vi "SW_Check_segments_parameters_2.vi"(3 "Error In":errorcluster, 5 "Geometry in":T1 {"Cage type" items=["Round", "Square", "Donut-maze", "T-maze", "Sociability maze", ""]}) -> (0 "Error Out":errorcluster, 1 "Segmentation out":T4={"CENTER"={"Radius, mm CENTER"=30}, "MIDFIELD"={"Radius, mm MIDFIELD"=75, "N segments MIDFIELD"=2, "Starting angle MIDFIELD"=0}, "BORDER"={"N segments BORDER"=4, "Starting angle BORDER"=0}} {"BORDER"."N segments BORDER" min=1 max=12; "MIDFIELD"."N segments MIDFIELD" max=8; "CENTER"."Radius, mm CENTER" min=5 step=1}, 2 "Geometry out":T1 {"Cage type" items=["Round", "Square", "Donut-maze", "T-maze", "Sociability maze", ""]})   [LabVIEW 2018, in "Tracker.lvlib"]
uses:
  Tracker.lvlib
  Controls/CTL_Cage_radial_segmentation.ctl
  Controls/CTL_Segmented_plot_parameters_2.ctl
  Libraries/Cage Diagram/Typedefs/CTL_Cage_type.ctl
  Controls/CTL_Cage_all_segmentation_params_set.ctl
  Controls/CTL_Segmented_plot_parameters_2_(round_d1).ctl
  Common_Resources.lvlib
  Libraries/Cage Diagram/Cage Diagram.lvlib
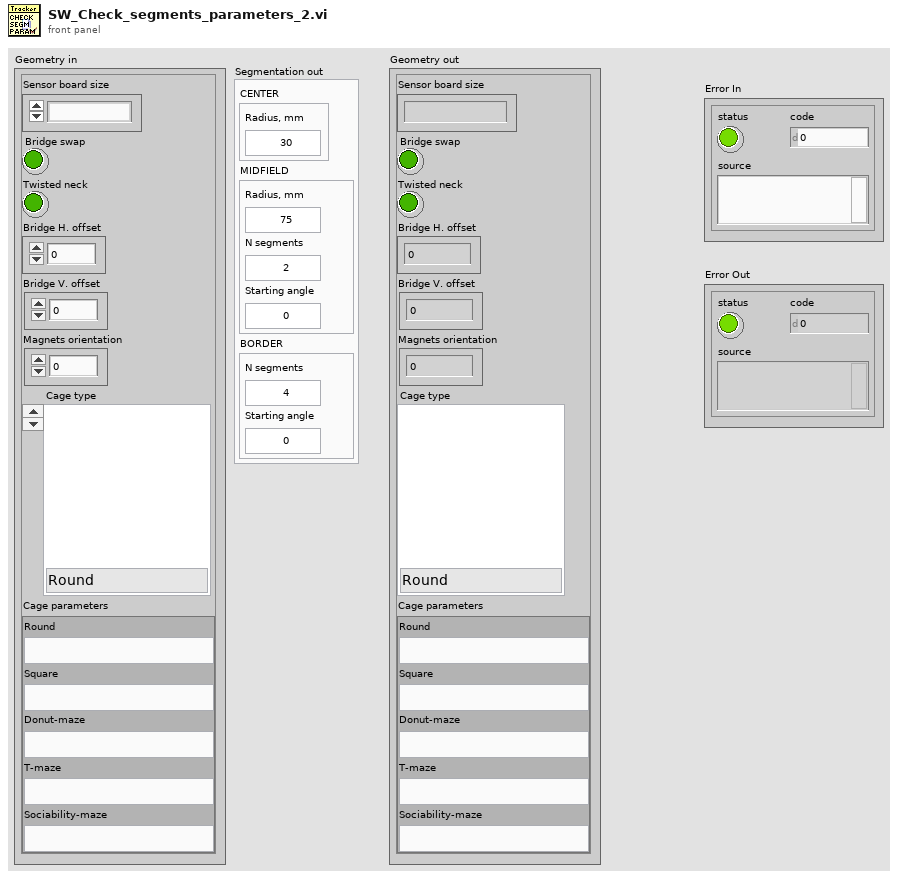
[diagram p1: front panel]
types:
  T1 = typedef "Common_Resources.lvlib/CTL_Segmented_plot_parameters_2.ctl" = cluster{"Sensor board size":enum16{"", "Large"}, "Bridge swap":bool, "Twisted neck":bool, "Bridge H. offset":sgl, "Bridge V. offset":sgl, "Magnets orientation":sgl, "Cage type":T2, "Cage parameters":T3}
  T2 = typedef "Cage Diagram.lvlib/CTL_Cage_type.ctl" = u16
  T3 = typedef "Common_Resources.lvlib/CTL_Cage_all_segmentation_params_set.ctl" = cluster{"Round":variant, "Square":variant, "Donut-maze":variant, "T-maze":variant, "Sociability-maze":variant}
  T4 = typedef "Common_Resources.lvlib/CTL_Cage_radial_segmentation.ctl" = cluster{"CENTER":cluster{"Radius, mm CENTER":u16}, "MIDFIELD":cluster{"Radius, mm MIDFIELD":u16, "N segments MIDFIELD":u8, "Starting angle MIDFIELD":i16}, "BORDER":cluster{"N segments BORDER":u8, "Starting angle BORDER":i16}}
  T5 = typedef "Common_Resources.lvlib/CTL_Segmented_plot_parameters_2_(round_d1).ctl" = cluster{"Cage diameter, mm":u16, "Starting angle BORDER":i16, "Starting angle MIDFIELD":i16, "Radius, mm MIDFIELD":u16, "Radius, mm CENTER":u16, "N segments BORDER":u8, "N segments MIDFIELD":u8, "R-gap, mm":sgl}
  T6 = cluster{"Radius, mm MIDFIELD":u16, "N segments MIDFIELD":u8, "Starting angle MIDFIELD":i16}
  T7 = cluster{"N segments BORDER":u8, "Starting angle BORDER":i16}
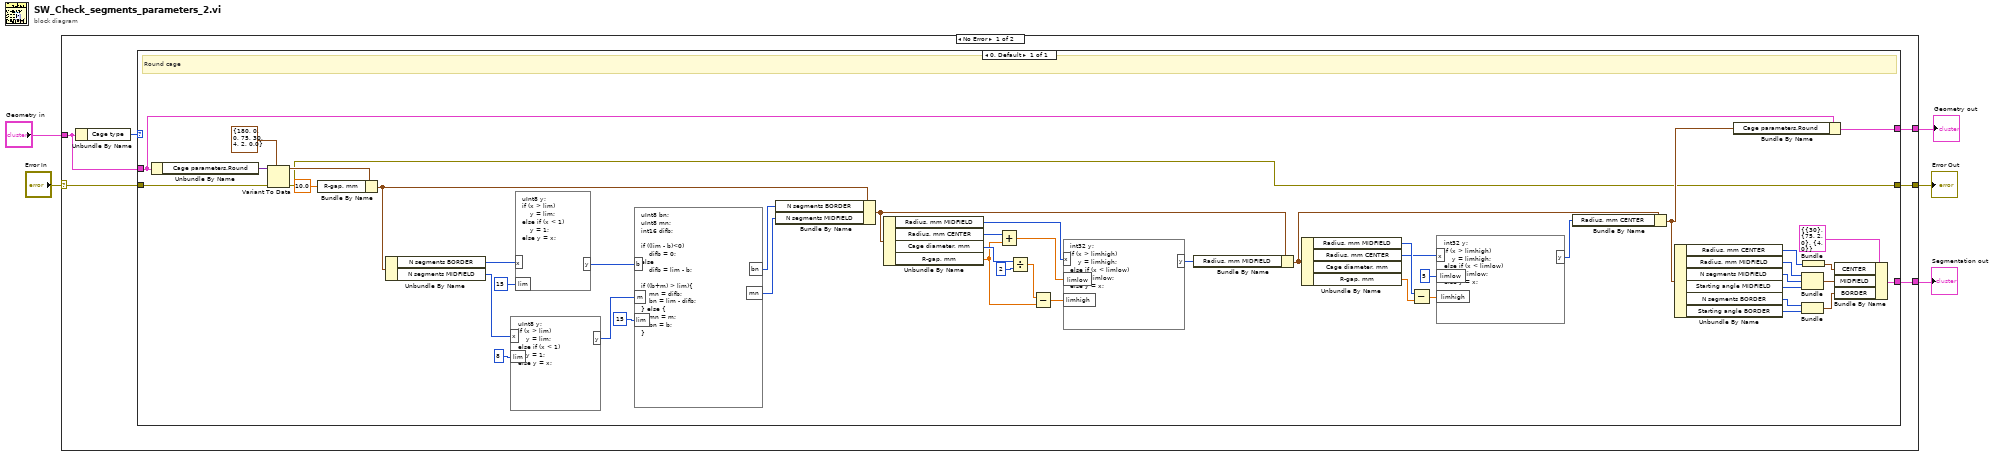
[diagram p0: block diagram]
diagram:
  n1 = case shown="No Error" "Error In" {
    selector: "Error In" -> [w8 w60]
    tunnel: [w11 _] -> w5
    tunnel: [w6 w60] -> w3
    tunnel: "Geometry in" -> [w9 w59]
    tunnel: [w7 w59] -> w1
    frame No Error {
      n2 = Unbundle By Name(w9) -> ("Cage type"=w10:T2)
      n3 = case shown="0, Default" w10 {
        tunnel: [w20] -> w11
        tunnel: w9 -> [w16]
        tunnel: w8 -> [w18]
        tunnel: [w13] -> w7
        tunnel: [w12] -> w6
        frame 0, Default {
          # "Round cage"
          n4 = Unbundle By Name(w16) -> ("Cage parameters.Round"=w19:variant)
          n5 = Variant To Data(error in=w18, type=T5 {"Cage diameter, mm"=180, "Starting angle BORDER"=0, "Starting angle MIDFIELD"=0, "Radius, mm MIDFIELD"=75, "Radius, mm CENTER"=30, "N segments BORDER"=4, "N segments MIDFIELD"=2, "R-gap, mm"=0.0} ("Radial segmentation parameters"), Variant=w19) -> (data=w17:T5, error out=w12:errorcluster)
          n6 = Bundle By Name(cluster=w17, "R-gap, mm"=sgl 10.0) -> (w43:T5)
          n7 = Unbundle By Name(w43) -> ("N segments BORDER"=w47:u8, "N segments MIDFIELD"=w46:u8)
          n8 = formula code="uInt8 y;\nif (x > lim)\n    y = lim;\nelse if (x < 1)\n    y = 1;\nelse y = x;"("x"=w46, "lim"=u8 8 ("input variable")) -> ("y"=w49:u8)
          n9 = formula code="uInt8 y;\nif (x > lim)\n    y = lim;\nelse if (x < 1)\n    y = 1;\nelse y = x;"("x"=w47, "lim"=u8 15 ("input variable")) -> ("y"=w50:u8)
          n10 = formula code="uInt8 bn;\nuInt8 mn;\nint16 difb;\n\nif ((lim - b)<0) \n    difb = 0;\nelse\n    difb = lim - b;\n\nif ((b+m) > lim){\n    mn = difb;\n    bn = lim - difb;\n} else {\n    mn = m;\n    bn = b;\n}"("b"=w50, "m"=w49, "lim"=u8 15 ("input variable")) -> ("bn"=w45:u8, "mn"=w44:u8)
          n11 = Bundle By Name(cluster=w43, "N segments BORDER"=w45, "N segments MIDFIELD"=w44) -> (w38:T5)
          n12 = Unbundle By Name(w38) -> ("Radius, mm MIDFIELD"=w41:u16, "Radius, mm CENTER"=w40:u16, "Cage diameter, mm"=w39:u16, "R-gap, mm"=w31:sgl)
          n13 = Add(x=w40, y=w31) -> (x+y=w53:sgl)
          n14 = Divide(x=w39, y=u16 2) -> (x/y=w55:dbl)
          n15 = Subtract(x=w55, y=w31) -> (x-y=w54:dbl)
          n16 = formula code="int32 y;\nif (x > limhigh)\n    y = limhigh;\nelse if (x < limlow)\n    y = limlow;\nelse y = x;"("x"=w41, "limlow"=w53, "limhigh"=w54) -> ("y"=w37:i32)
          n17 = Bundle By Name(cluster=w38, "Radius, mm MIDFIELD"=w37) -> (w33:T5)
          n18 = Unbundle By Name(w33) -> ("Radius, mm MIDFIELD"=w36:u16, "Radius, mm CENTER"=w35:u16, "R-gap, mm"=w34:sgl)  [unwired: 1 out]
          n19 = Subtract(x=w36, y=w34) -> (x-y=w51:sgl)
          n20 = formula code="int32 y;\nif (x > limhigh)\n    y = limhigh;\nelse if (x < limlow)\n    y = limlow;\nelse y = x;"("x"=w35, "limlow"=5 ("input variable"), "limhigh"=w51) -> ("y"=w32:i32)
          n21 = Bundle By Name(cluster=w33, "Radius, mm CENTER"=w32) -> (w14:T5)
          n22 = Unbundle By Name(w14) -> ("Radius, mm CENTER"=w30:u16, "Radius, mm MIDFIELD"=w28:u16, "N segments MIDFIELD"=w27:u8, "Starting angle MIDFIELD"=w26:i16, "N segments BORDER"=w24:u8, "Starting angle BORDER"=w23:i16)
          n23 = Bundle By Name(cluster=w16, "Cage parameters.Round"=w14) -> (w13:T1)
          n24 = Bundle("Radius, mm MIDFIELD"=w28, "N segments MIDFIELD"=w27, "Starting angle MIDFIELD"=w26) -> (w25:T6)  [unwired: 1 in]
          n25 = Bundle("N segments BORDER"=w24, "Starting angle BORDER"=w23) -> (w22:T7)  [unwired: 1 in]
          n26 = Bundle("Radius, mm CENTER"=w30) -> (w29:cluster{"Radius, mm CENTER":u16})  [unwired: 1 in]
          n27 = Bundle By Name(cluster=T4 {"CENTER"={"Radius, mm CENTER"=30}, "MIDFIELD"={"Radius, mm MIDFIELD"=75, "N segments MIDFIELD"=2, "Starting angle MIDFIELD"=0}, "BORDER"={"N segments BORDER"=4, "Starting angle BORDER"=0}} ("Cage radial segmentation"), "CENTER"=w29, "MIDFIELD"=w25, "BORDER"=w22) -> (w20:T4)
        }
      }
    }
    frame Error {
    }
  }
  "Error Out" <- w3
  "Segmentation out" <- w5
  "Geometry out" <- w1
